vi "Baseline_remove_single.vi"(9 "B array":dbl[](array[numeric]), 10 "I(B) in":dbl[](array[numeric]), 11 "B0":dbl) -> (2 "mean 1":dbl format="%0.2f", 3 "BaselineSubtracted I(B)":dbl[](array[numeric]))   [LabVIEW 2015]
uses:
  <vilib>/Analysis/baseanly.llb/Mean (DBL).vi
  <vilib>/Analysis/NI_AALBase.lvlib
panel:
  out "I(B) out":cluster{"B array":dbl[], dbl[]}(graph)
  out "Ending":cluster{dbl[], dbl[]}(graph)
  out "I(B) in":cluster{"B array":dbl[], "I(B) in":dbl[]}(graph)
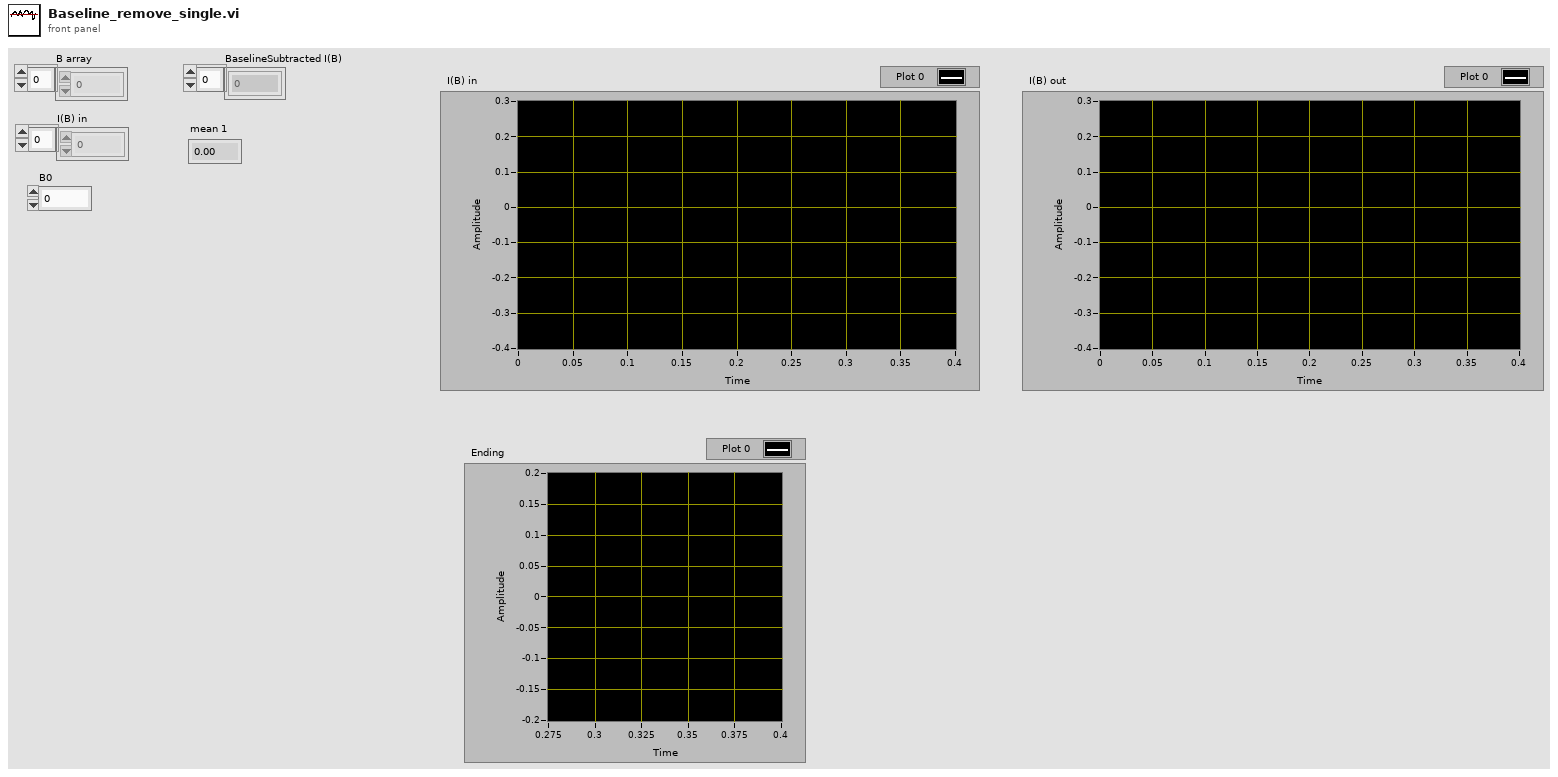
[diagram p1: front panel]
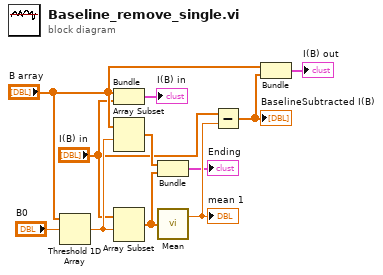
[diagram p0: block diagram]
diagram:
  n1 = Threshold 1D Array(2:"B0", 3:"B array") -> (0:w7:dbl)  [unwired: 1 in]
  n2 = Bundle("B array"="B array", "I(B) in"="I(B) in") -> (→"I(B) in":cluster{"B array":dbl[], "I(B) in":dbl[]})  [unwired: 1 in]
  n3 = Array Subset(array="B array", index=w7) -> (w8:dbl[])  [unwired: 1 in]
  n4 = Array Subset(array="I(B) in", index=w7) -> (w9:dbl[])  [unwired: 1 in]
  n5 = Bundle(w8, w9) -> (→"Ending":cluster{dbl[], dbl[]})  [unwired: 1 in]
  n6 = call-poly <vilib>:"Mean.vi"("X"=w9) -> ("mean"=w10:dbl)  [unwired: 1 out]
  "mean 1" <- w10
  n7 = Subtract(x="I(B) in", y=w10) -> (x-y=w11:dbl[])
  "BaselineSubtracted I(B)" <- w11
  n8 = Bundle("B array"="B array", w11) -> (→"I(B) out":cluster{"B array":dbl[], dbl[]})  [unwired: 1 in]
